vi "Pre-Actor.vi"(8 "error in":errorcluster, 11 "Electronic Load in":refnum<class "Electronic Load.lvclass">) -> (0 "error out":errorcluster, 3 "Electronic Load out":refnum<class "Electronic Load.lvclass">)   [LabVIEW 2019, in "Electronic Load.lvlib" / "Electronic Load.lvclass"]
doc: "This override VI is to provide the means for children classes to perform application specific post launch initialization functions that must be performed *prior* to calling the actor. \n\n***DO NOT USE THE CHECK FOR FAULT ROUTINE HERE***"
uses:
  Library/Electronic Load.lvclass
  C:/Users/Public/Documents/Development/builds/Instruments/Instruments.lvlibp/Library/Instruments.lvclass
  Library/Electronic Load.lvclass/Electronic Load.ctl
  Private/GUI/Read Trigger_TargetsRef.vi
  Accessors/Read Available Channels.vi
  builds/Instruments/Instruments.lvlibp/Accessors/Read Graph_Ref.vi
  builds/Instruments/Instruments.lvlibp/Accessors/Read Snapshot Refnum.vi
  builds/Instruments/Instruments.lvlibp/Library/Instruments.lvclass
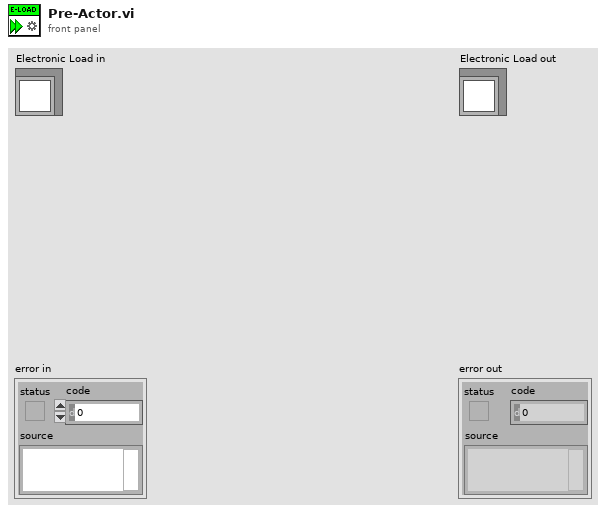
[diagram p1: front panel]
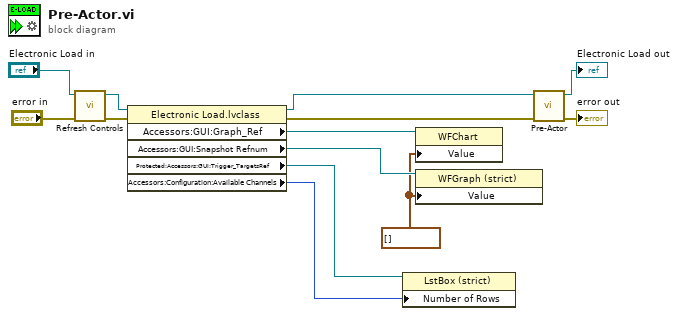
[diagram p0: block diagram]
diagram:
  w3 = waveform(dbl)[] [] ("Value")
  n1 = call "Refresh Controls.vi"("error in"="error in", "Electronic Load in"="Electronic Load in") -> ("error out"=w9:errorcluster, "Electronic Load out"=w8:refnum<class "Electronic Load.lvclass">)  [unwired: 8 in]
  n2 = property class="Electronic Load.lvclass"(reference=w8, error in=w9) -> (reference out=w7:refnum<class "Electronic Load.lvclass">, error out=w6:errorcluster, "Accessors:GUI:Graph_Ref"=w5:refnum<vi>, "Accessors:GUI:Snapshot Refnum"=w4:refnum<vi>, "Protected:Accessors:GUI:Trigger_TargetsRef"=w2:refnum<vi>, "Accessors:Configuration:Available Channels"=w1:i32)
  n3 = property class="LstBox (strict)"(reference=w2, "Number of Rows"=w1) -> ()  [unwired: 1 in, 2 out]
  n4 = property class="WFChart"(reference=w5, "Value"=w3) -> ()  [unwired: 1 in, 2 out]
  n5 = property class="WFGraph (strict)"(reference=w4, "Value"=w3) -> ()  [unwired: 1 in, 2 out]
  n6 = call-parent "Pre-Actor.vi"("error in (no error)"=w6, "Instruments in"=w7) -> ("error out"=→"error out":errorcluster, "Instruments out"=→"Electronic Load out":refnum<class "Electronic Load.lvclass">)  [unwired: 8 in]
